vi "parseIDLFile.vi"(8 "error in (no error)":errorcluster, 10 "idlFilepath":path, 11 "IDLFile in":refnum<class "IDLFile.lvclass">) -> (0 "error out":errorcluster, 3 "IDLFile out":refnum<class "IDLFile.lvclass">)   [LabVIEW 2016, in "IDLFile.lvclass"]
uses:
  IDLFile.lvclass
  IDLFile.lvclass/IDLFile.ctl
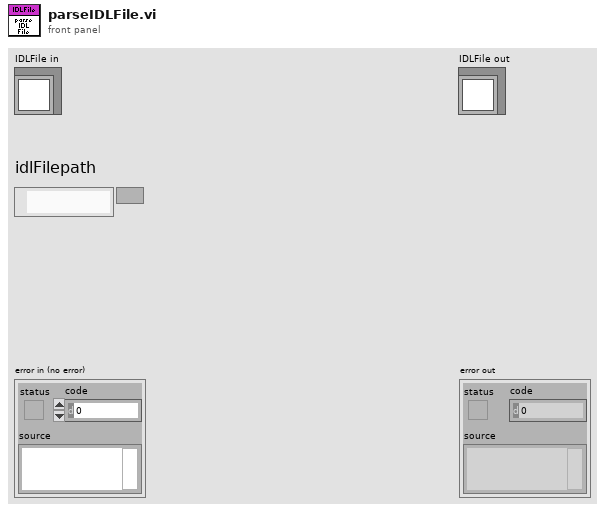
[diagram p1: front panel]
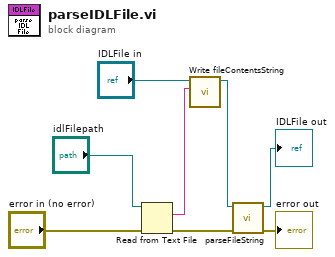
[diagram p0: block diagram]
diagram:
  n1 = Read from Text File(file (use dialog)="idlFilepath", error in="error in (no error)") -> (text=w2:string, error out=w6:errorcluster)  [unwired: 2 in, 2 out]
  n2 = call "Write fileContentsString.vi"("fileContentsString"=w2, "IDLFile in"="IDLFile in") -> ("IDLFile out"=w1:refnum<class "IDLFile.lvclass">)  [unwired: 9 in]
  n3 = call "parseFileString.vi"("error in (no error)"=w6, "IDLFile in"=w1) -> ("error out"=→"error out":errorcluster, "IDLFile out"=→"IDLFile out":refnum<class "IDLFile.lvclass">)  [unwired: 8 in]
